vi "Manual Test.vi"() -> ()   [LabVIEW 2020, in "driver_flodx_pressure.lvlib"]
uses:
  <instrlib>/RxnRover/FloDx Pressure Driver/driver_flodx_pressure.lvlib
panel:
  out "Raw Response":string
  in  "Set Units Num":u8 max=2
  in  "Set Max Ambient Pressure Num":dbl
  in  "Set Max Sensitivity Num":dbl
  in  "Set Ambient To Current Pressure":bool
  in  "Set Ambient Pressure":bool
  in  "Set Max Sensitivity":bool
  in  "Set Units":bool
  in  "Print Max Sensitivity":bool
  in  "Print Units":bool
  in  "Print Temperature":bool
  in  "Print Absolute Pressure":bool
  in  "Print Ambient Pressure":bool
  in  "Print Gauge Pressure":bool
  out "Units(0-kPa,1-PSI,2-BAR)":u8
  out "Max Sensitivity":sgl
  out "Temperature":sgl
  out "Absolute Pressure":sgl
  out "Ambient Pressure":sgl
  out "Gauge Pressure":sgl
  in  "Address":u8
  in  "error in (no error)":errorcluster
  in  "VISA resource name":refnum<visa-resource-name>
  out "error out":errorcluster
  out "VISA resource name out":refnum<visa-resource-name>
  in  "Close Communication with Device":bool
  in  "Initialize  For Test DO THIS BEFORE RUNNING ANY TESTS":bool
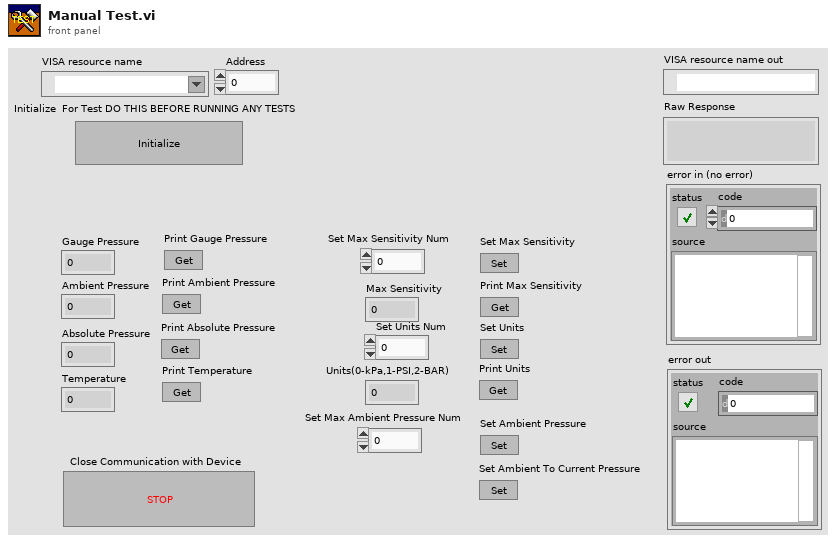
[diagram p1: front panel]
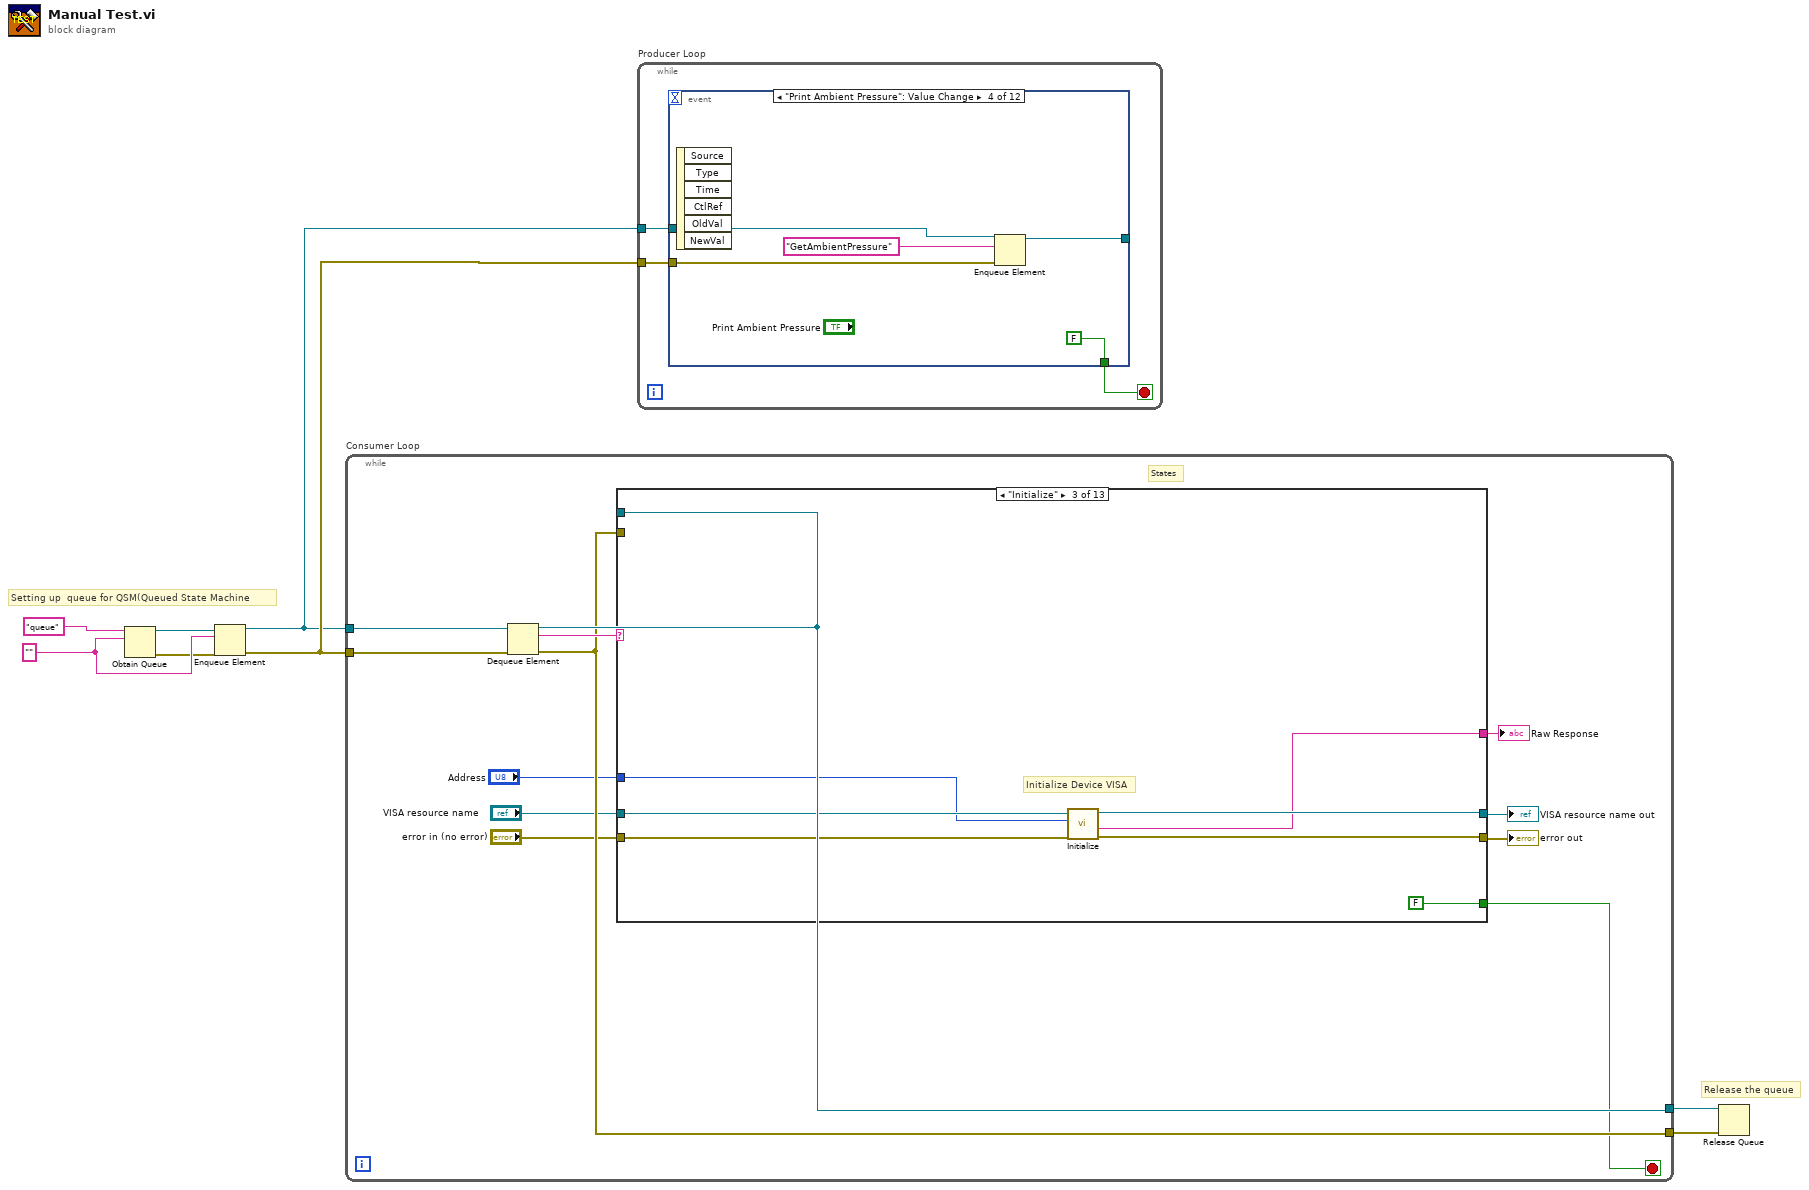
[diagram p0: block diagram]
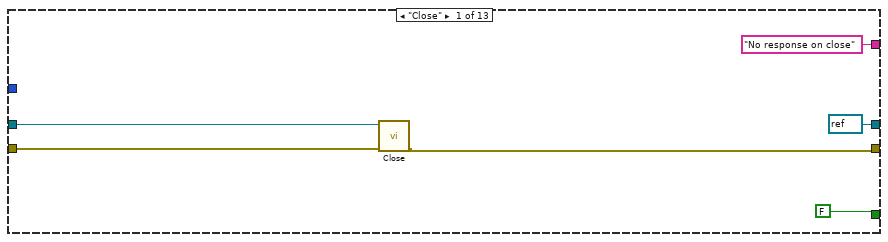
[diagram p2: hidden frame]
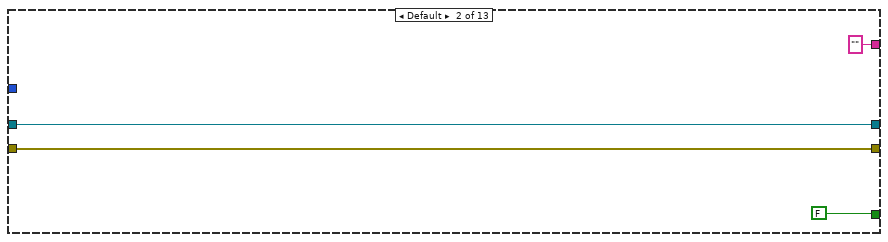
[diagram p3: hidden frame]
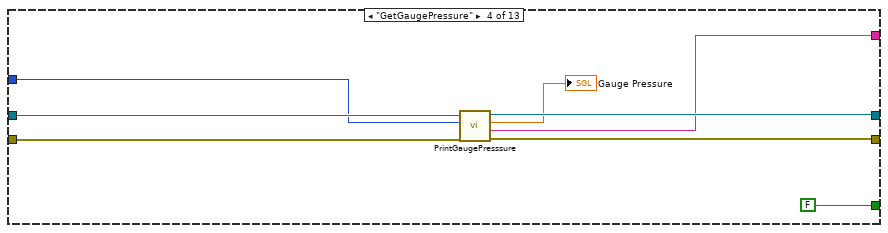
[diagram p4: hidden frame]
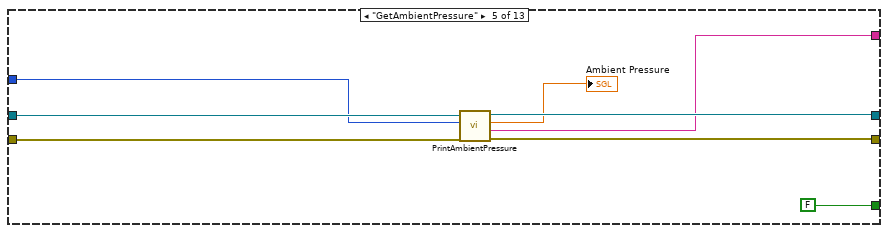
[diagram p5: hidden frame]
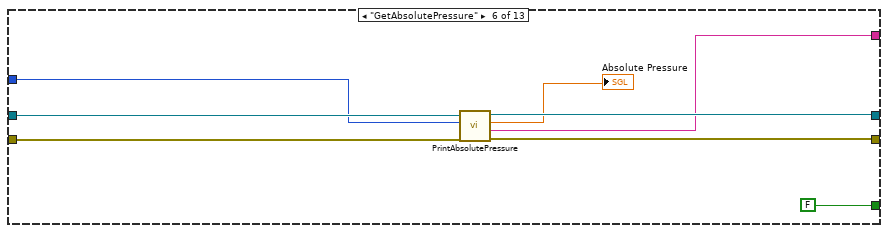
[diagram p6: hidden frame]
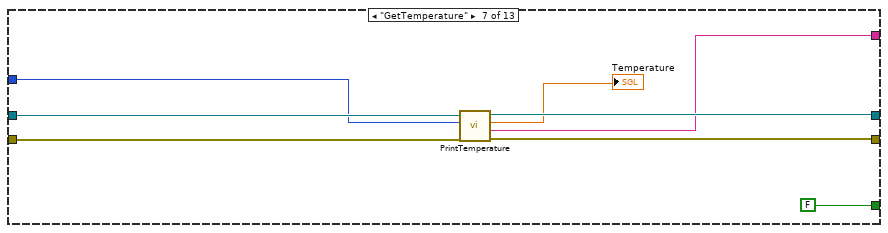
[diagram p7: hidden frame]
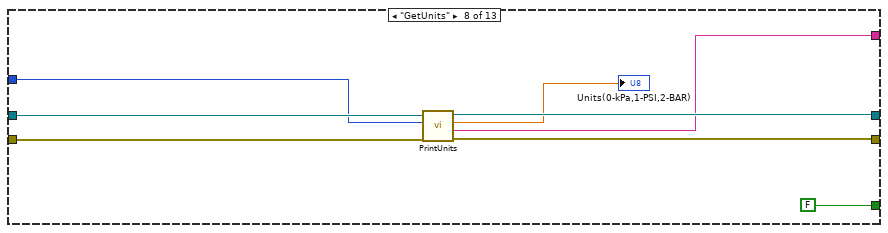
[diagram p8: hidden frame]
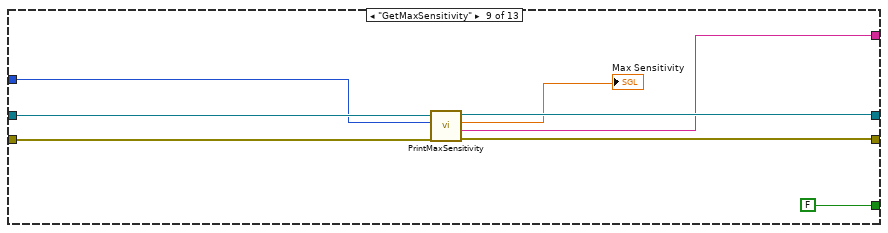
[diagram p9: hidden frame]
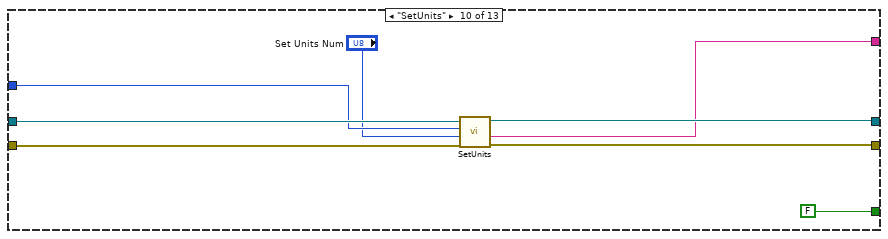
[diagram p10: hidden frame]
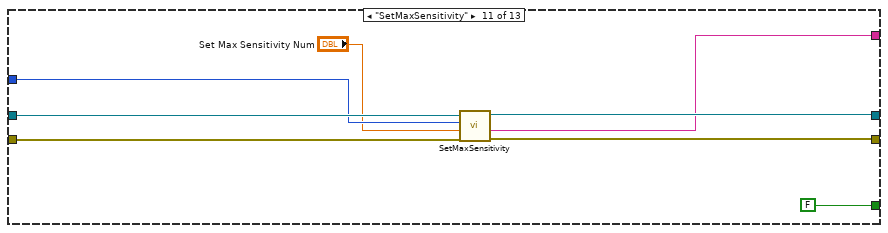
[diagram p11: hidden frame]
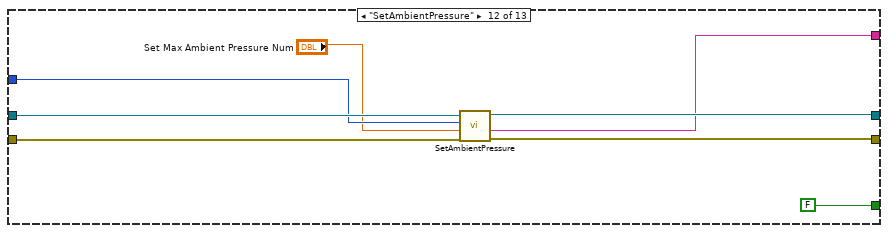
[diagram p12: hidden frame]
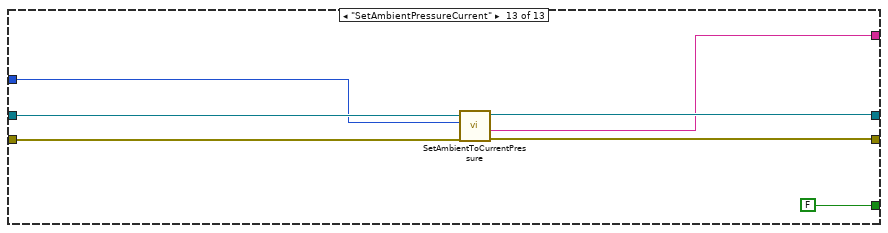
[diagram p13: hidden frame]
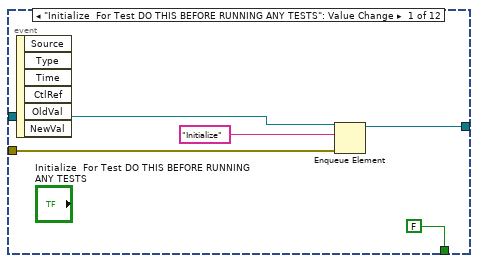
[diagram p14: hidden frame]
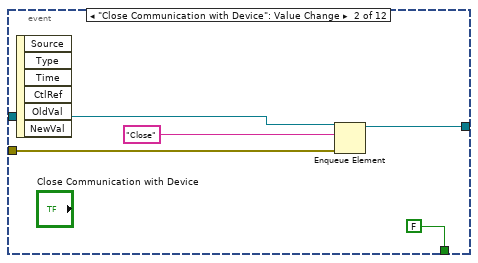
[diagram p15: hidden frame]
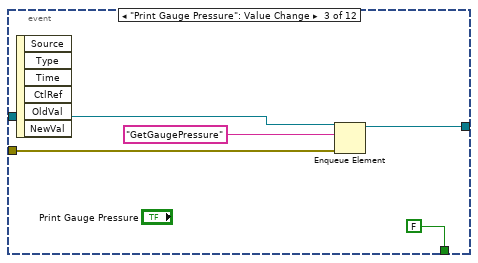
[diagram p16: hidden frame]
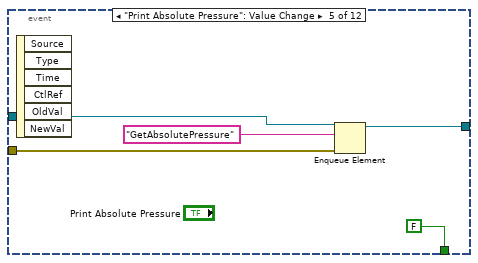
[diagram p17: hidden frame]
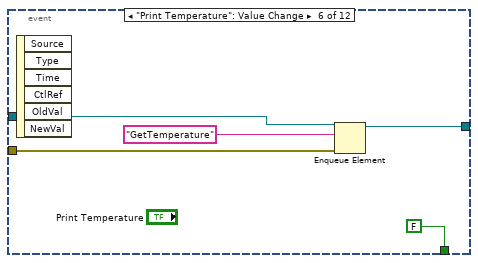
[diagram p18: hidden frame]
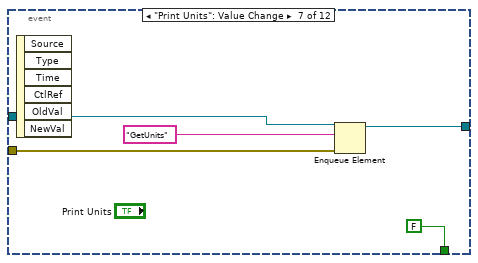
[diagram p19: hidden frame]
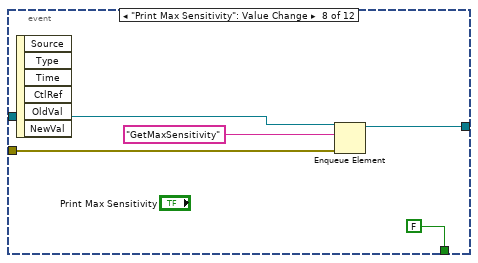
[diagram p20: hidden frame]
diagram:
  w7 = ""
  # "Release the queue"
  # "Setting up  queue for QSM(Queued State Machine"
  n1 = Obtain Queue(name (unnamed)="queue", element data type=w7) -> (queue out=w6:refnum<queue>, error out=w5:errorcluster)  [unwired: 3 in, 1 out]
  n2 = Enqueue Element(queue=w6, element=w7, error in (no error)=w5) -> (queue out=w1:refnum<queue>, error out=w2:errorcluster)  [unwired: 1 in, 1 out]
  n3 = while "Consumer Loop" {
    tunnel: [w17] -> w4
    tunnel: [w16] -> w3
    tunnel: w2 -> [w20]
    tunnel: w1 -> [w19]
    stop <- w11 stop-if-true
    # "States"
    n4 = Dequeue Element(queue=w19, error in (no error)=w20) -> (queue out=w17:refnum<queue>, element=w18:string, error out=w16:errorcluster)  [unwired: 1 in, 1 out]
    n5 = case shown="\"Initialize\"" w18 {
      tunnel: w17 -> [_ _ _ _ _ _ _ _ _ _ _ _ _]
      tunnel: w16 -> [_ _ _ _ _ _ _ _ _ _ _ _ _]
      tunnel: "VISA resource name" -> [w22 w30 w33 w41 w49 w57 w65 w73 w81 w89 w97 w105 w112]
      tunnel: "error in (no error)" -> [w23 w29 w34 w42 w50 w58 w66 w74 w82 w90 w98 w106 w113]
      tunnel: [refnum<visa-resource-name> refnum ("VISA resource name out") w30 w36 w44 w52 w60 w68 w76 w84 w92 w100 w108 w115] -> w13
      tunnel: [w24 w29 w35 w43 w51 w59 w67 w75 w83 w91 w99 w107 w114] -> w12
      tunnel: [FALSE FALSE FALSE FALSE FALSE FALSE FALSE FALSE FALSE FALSE FALSE FALSE FALSE] -> w11
      tunnel: "Address" -> [_ _ w32 w40 w48 w56 w64 w72 w80 w88 w96 w104 w111]
      tunnel: ["No response on close" ("Raw Response") "" ("Raw Response") w31 w38 w47 w55 w63 w71 w79 w87 w95 w103 w110] -> w9
      frame "Close" {
        n6 = call <instrlib>:"Close.vi"("error in (no error)"=w23, "VISA resource name"=w22) -> ("error out"=w24:errorcluster)  [unwired: 9 in]
      }
      frame Default {
      }
      frame "Initialize" {
        # "Initialize Device VISA"
        n7 = call <instrlib>:"Initialize.vi"("error in (no error)"=w34, "Address"=w32, "VISA resource name"=w33) -> ("error out"=w35:errorcluster, "Raw Response"=w31:string, "VISA resource name out"=w36:refnum<visa-resource-name>)  [unwired: 6 in]
      }
      frame "GetGaugePressure" {
        n8 = call <instrlib>:"PrintGaugePresssure.vi"("error in (no error)"=w42, "Address"=w40, "VISA resource name"=w41) -> ("error out"=w43:errorcluster, "Raw Response"=w38:string, "Print Gauge Pressure"=→"Gauge Pressure":dbl, "VISA resource name out"=w44:refnum<visa-resource-name>)  [unwired: 5 in]
      }
      frame "GetAmbientPressure" {
        n9 = call <instrlib>:"PrintAmbientPressure.vi"("error in (no error)"=w50, "Address"=w48, "VISA resource name"=w49) -> ("error out"=w51:errorcluster, "Raw Response"=w47:string, "Ambient Pressure"=→"Ambient Pressure":dbl, "VISA resource name out"=w52:refnum<visa-resource-name>)  [unwired: 5 in]
      }
      frame "GetAbsolutePressure" {
        n10 = call <instrlib>:"PrintAbsolutePressure.vi"("error in (no error)"=w58, "Address"=w56, "VISA resource name"=w57) -> ("error out"=w59:errorcluster, "Raw Response"=w55:string, "Abs. Pressure"=→"Absolute Pressure":dbl, "VISA resource name out"=w60:refnum<visa-resource-name>)  [unwired: 5 in]
      }
      frame "GetTemperature" {
        n11 = call <instrlib>:"PrintTemperature.vi"("error in (no error)"=w66, "Address"=w64, "VISA resource name"=w65) -> ("error out"=w67:errorcluster, "Raw Response"=w63:string, "Temperature"=→"Temperature":dbl, "VISA resource name out"=w68:refnum<visa-resource-name>)  [unwired: 5 in]
      }
      frame "GetUnits" {
        n12 = call <instrlib>:"PrintUnits.vi"("error in (no error)"=w74, "Address"=w72, "VISA resource name"=w73) -> ("error out"=w75:errorcluster, "Raw Response"=w71:string, "Units(0-Kpa,1-PSI,2-BAR)"=→"Units(0-kPa,1-PSI,2-BAR)":dbl, "VISA resource name out"=w76:refnum<visa-resource-name>)  [unwired: 5 in]
      }
      frame "GetMaxSensitivity" {
        n13 = call <instrlib>:"PrintMaxSensitivity.vi"("error in (no error)"=w82, "Address"=w80, "VISA resource name"=w81) -> ("error out"=w83:errorcluster, "Raw Response"=w79:string, "Max Sensitivity"=→"Max Sensitivity":dbl, "VISA resource name out"=w84:refnum<visa-resource-name>)  [unwired: 5 in]
      }
      frame "SetUnits" {
        n14 = call <instrlib>:"SetUnits.vi"("error in (no error)"=w90, "Unit(0-kPa,1-PSI,2-BAR)"="Set Units Num", "Address"=w88, "VISA resource name"=w89) -> ("error out"=w91:errorcluster, "Raw Response"=w87:string, "VISA resource name out"=w92:refnum<visa-resource-name>)  [unwired: 5 in]
      }
      frame "SetMaxSensitivity" {
        n15 = call <instrlib>:"SetMaxSensitivity.vi"("error in (no error)"=w98, "Max Sensitivity"="Set Max Sensitivity Num", "Address"=w96, "VISA resource name"=w97) -> ("error out"=w99:errorcluster, "Raw Response"=w95:string, "VISA resource name out"=w100:refnum<visa-resource-name>)  [unwired: 5 in]
      }
      frame "SetAmbientPressure" {
        n16 = call <instrlib>:"SetAmbientPressure.vi"("error in (no error)"=w106, "Ambient Pressure"="Set Max Ambient Pressure Num", "Address"=w104, "VISA resource name"=w105) -> ("error out"=w107:errorcluster, "Raw Response"=w103:string, "VISA resource name out"=w108:refnum<visa-resource-name>)  [unwired: 5 in]
      }
      frame "SetAmbientPressureCurrent" {
        n17 = call <instrlib>:"SetAmbientToCurrentPressure.vi"("error in (no error)"=w113, "Address"=w111, "VISA resource name"=w112) -> ("error out"=w114:errorcluster, "Raw Response"=w110:string, "VISA resource name out"=w115:refnum<visa-resource-name>)  [unwired: 6 in]
      }
    }
    "error out" <- w12
    "VISA resource name out" <- w13
    "Raw Response" <- w9
  }
  n18 = while "Producer Loop" {
    tunnel: w2 -> [w119]
    tunnel: w1 -> [w118]
    stop <- w117 stop-if-true
    n19 = event shown="[3] \"Print Ambient Pressure\": Value Change" {
      selector: _ -> [_ _ _ _ _ _ _ _ _ _ _ _]
      dyn-events: _ -> [_ _ _ _ _ _ _ _ _ _ _ _]
      timeout: _ -> [_ _ _ _ _ _ _ _ _ _ _ _]
      tunnel: w119 -> [w123 w128 w133 w138 w143 w148 w153 w158 w163 w168 w173 w178]
      tunnel: w118 -> [w122 w127 w132 w137 w142 w147 w152 w157 w162 w167 w172 w177]
      tunnel: [w121 w126 w131 w136 w141 w146 w151 w156 w161 w166 w171 w176] -> _
      tunnel: [FALSE FALSE FALSE FALSE FALSE FALSE FALSE FALSE FALSE FALSE FALSE FALSE] -> w117
      event "Initialize  For Test DO THIS BEFORE RUNNING ANY TESTS": Value Change {
        n20 = event-data() -> ()  [unwired: 1 in, 6 out]
        n21 = Enqueue Element(queue=w122, element="Initialize", error in (no error)=w123) -> (queue out=w121:refnum<queue>)  [unwired: 1 in, 2 out]
      }
      event "Close Communication with Device": Value Change {
        n22 = event-data() -> ()  [unwired: 1 in, 6 out]
        n23 = Enqueue Element(queue=w127, element="Close", error in (no error)=w128) -> (queue out=w126:refnum<queue>)  [unwired: 1 in, 2 out]
      }
      event "Print Gauge Pressure": Value Change {
        n24 = event-data() -> ()  [unwired: 1 in, 6 out]
        n25 = Enqueue Element(queue=w132, element="GetGaugePressure", error in (no error)=w133) -> (queue out=w131:refnum<queue>)  [unwired: 1 in, 2 out]
      }
      event "Print Ambient Pressure": Value Change {
        n26 = event-data() -> ()  [unwired: 1 in, 6 out]
        n27 = Enqueue Element(queue=w137, element="GetAmbientPressure", error in (no error)=w138) -> (queue out=w136:refnum<queue>)  [unwired: 1 in, 2 out]
      }
      event "Print Absolute Pressure": Value Change {
        n28 = event-data() -> ()  [unwired: 1 in, 6 out]
        n29 = Enqueue Element(queue=w142, element="GetAbsolutePressure", error in (no error)=w143) -> (queue out=w141:refnum<queue>)  [unwired: 1 in, 2 out]
      }
      event "Print Temperature": Value Change {
        n30 = event-data() -> ()  [unwired: 1 in, 6 out]
        n31 = Enqueue Element(queue=w147, element="GetTemperature", error in (no error)=w148) -> (queue out=w146:refnum<queue>)  [unwired: 1 in, 2 out]
      }
      event "Print Units": Value Change {
        n32 = event-data() -> ()  [unwired: 1 in, 6 out]
        n33 = Enqueue Element(queue=w152, element="GetUnits", error in (no error)=w153) -> (queue out=w151:refnum<queue>)  [unwired: 1 in, 2 out]
      }
      event "Print Max Sensitivity": Value Change {
        n34 = event-data() -> ()  [unwired: 1 in, 6 out]
        n35 = Enqueue Element(queue=w157, element="GetMaxSensitivity", error in (no error)=w158) -> (queue out=w156:refnum<queue>)  [unwired: 1 in, 2 out]
      }
      event "Set Units": Value Change {
        n36 = event-data() -> ()  [unwired: 1 in, 6 out]
        n37 = Enqueue Element(queue=w162, element="SetUnits", error in (no error)=w163) -> (queue out=w161:refnum<queue>)  [unwired: 1 in, 2 out]
      }
      event "Set Max Sensitivity": Value Change {
        n38 = event-data() -> ()  [unwired: 1 in, 6 out]
        n39 = Enqueue Element(queue=w167, element="SetMaxSensitivity", error in (no error)=w168) -> (queue out=w166:refnum<queue>)  [unwired: 1 in, 2 out]
      }
      event "Set Ambient Pressure": Value Change {
        n40 = event-data() -> ()  [unwired: 1 in, 6 out]
        n41 = Enqueue Element(queue=w172, element="SetAmbientPressure", error in (no error)=w173) -> (queue out=w171:refnum<queue>)  [unwired: 1 in, 2 out]
      }
      event "Set Ambient To Current Pressure": Value Change {
        n42 = event-data() -> ()  [unwired: 1 in, 6 out]
        n43 = Enqueue Element(queue=w177, element="SetAmbientPressureCurrent", error in (no error)=w178) -> (queue out=w176:refnum<queue>)  [unwired: 1 in, 2 out]
      }
    }
  }
  n44 = Release Queue(queue=w4, error in (no error)=w3) -> ()  [unwired: 1 in, 3 out]
